vi "dfd_Error Handlers (Multiple).vi"(8 "error in (no error)":errorcluster, 9 "error sources":i32[](array[numeric]), 10 "condition failed?":bool[](array[boolean])) -> (0 "error out":errorcluster)   [LabVIEW 2017, in "NI_DigFilterLicensed.lvlib"]
uses:
  <vilib>/addons/Digital Filter Design/NI_DigFilterLicensed.lvlib
  <vilib>/addons/Digital Filter Design/_Misc.llb/dfd_Error Cluster From Error Code (Scalar).vi
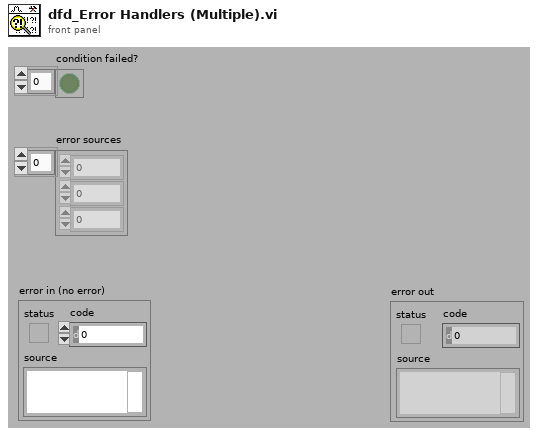
[diagram p1: front panel]
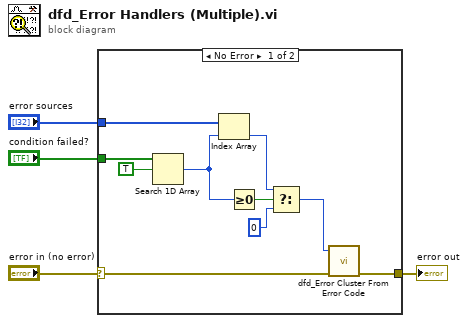
[diagram p0: block diagram]
diagram:
  n1 = case shown="No Error" "error in (no error)" {
    selector: "error in (no error)" -> [w10 w15]
    tunnel: "condition failed?" -> [w14 _]
    tunnel: "error sources" -> [w12 _]
    tunnel: [w11 w15] -> w2
    frame No Error {
      n2 = Search 1D Array(1D array=w14, element=TRUE) -> (index of element=w9:i32)  [unwired: 1 out]
      n3 = Index Array(array=w12, index=w9) -> (element=w7:i32)
      n4 = Greater Or Equal To 0?(x=w9) -> (x >= 0?=w8:bool)
      n5 = Select(t=w7, s=w8, f=0) -> (s? t:f=w5:i32)
      n6 = call-poly <vilib>:"dfd_Error Cluster From Error Code.vi"("error in (no error)"=w10, "error code (0)"=w5) -> ("error out"=w11:errorcluster)  [unwired: 9 out]
    }
    frame Error {
    }
  }
  "error out" <- w2
